vi "Att_Wobble.vi"(2 "Att Pos Z":refnum<vi>, 4 "Att Wobble End":dbl caption="End", 5 "Att Wobble Start":dbl caption="Start", 6 "Att Error":errorcluster, 7 "ourDLL":path, 8 "Att Wobble Stop2 2":refnum<vi>, 9 "Att DeviceHandle":u64) -> (0 "Att Error out":errorcluster, 3 "Att DeviceHandle out":u64)   [LabVIEW 2019]
panel:
  in  "Att Pos Z":dbl min=-500.0 max=3500.0 format="%#_7g"
  in  "Att Wobble Stop2":bool
  in  "Att Stop Wobble 2":bool
  in  "Att Stop Wobble":bool
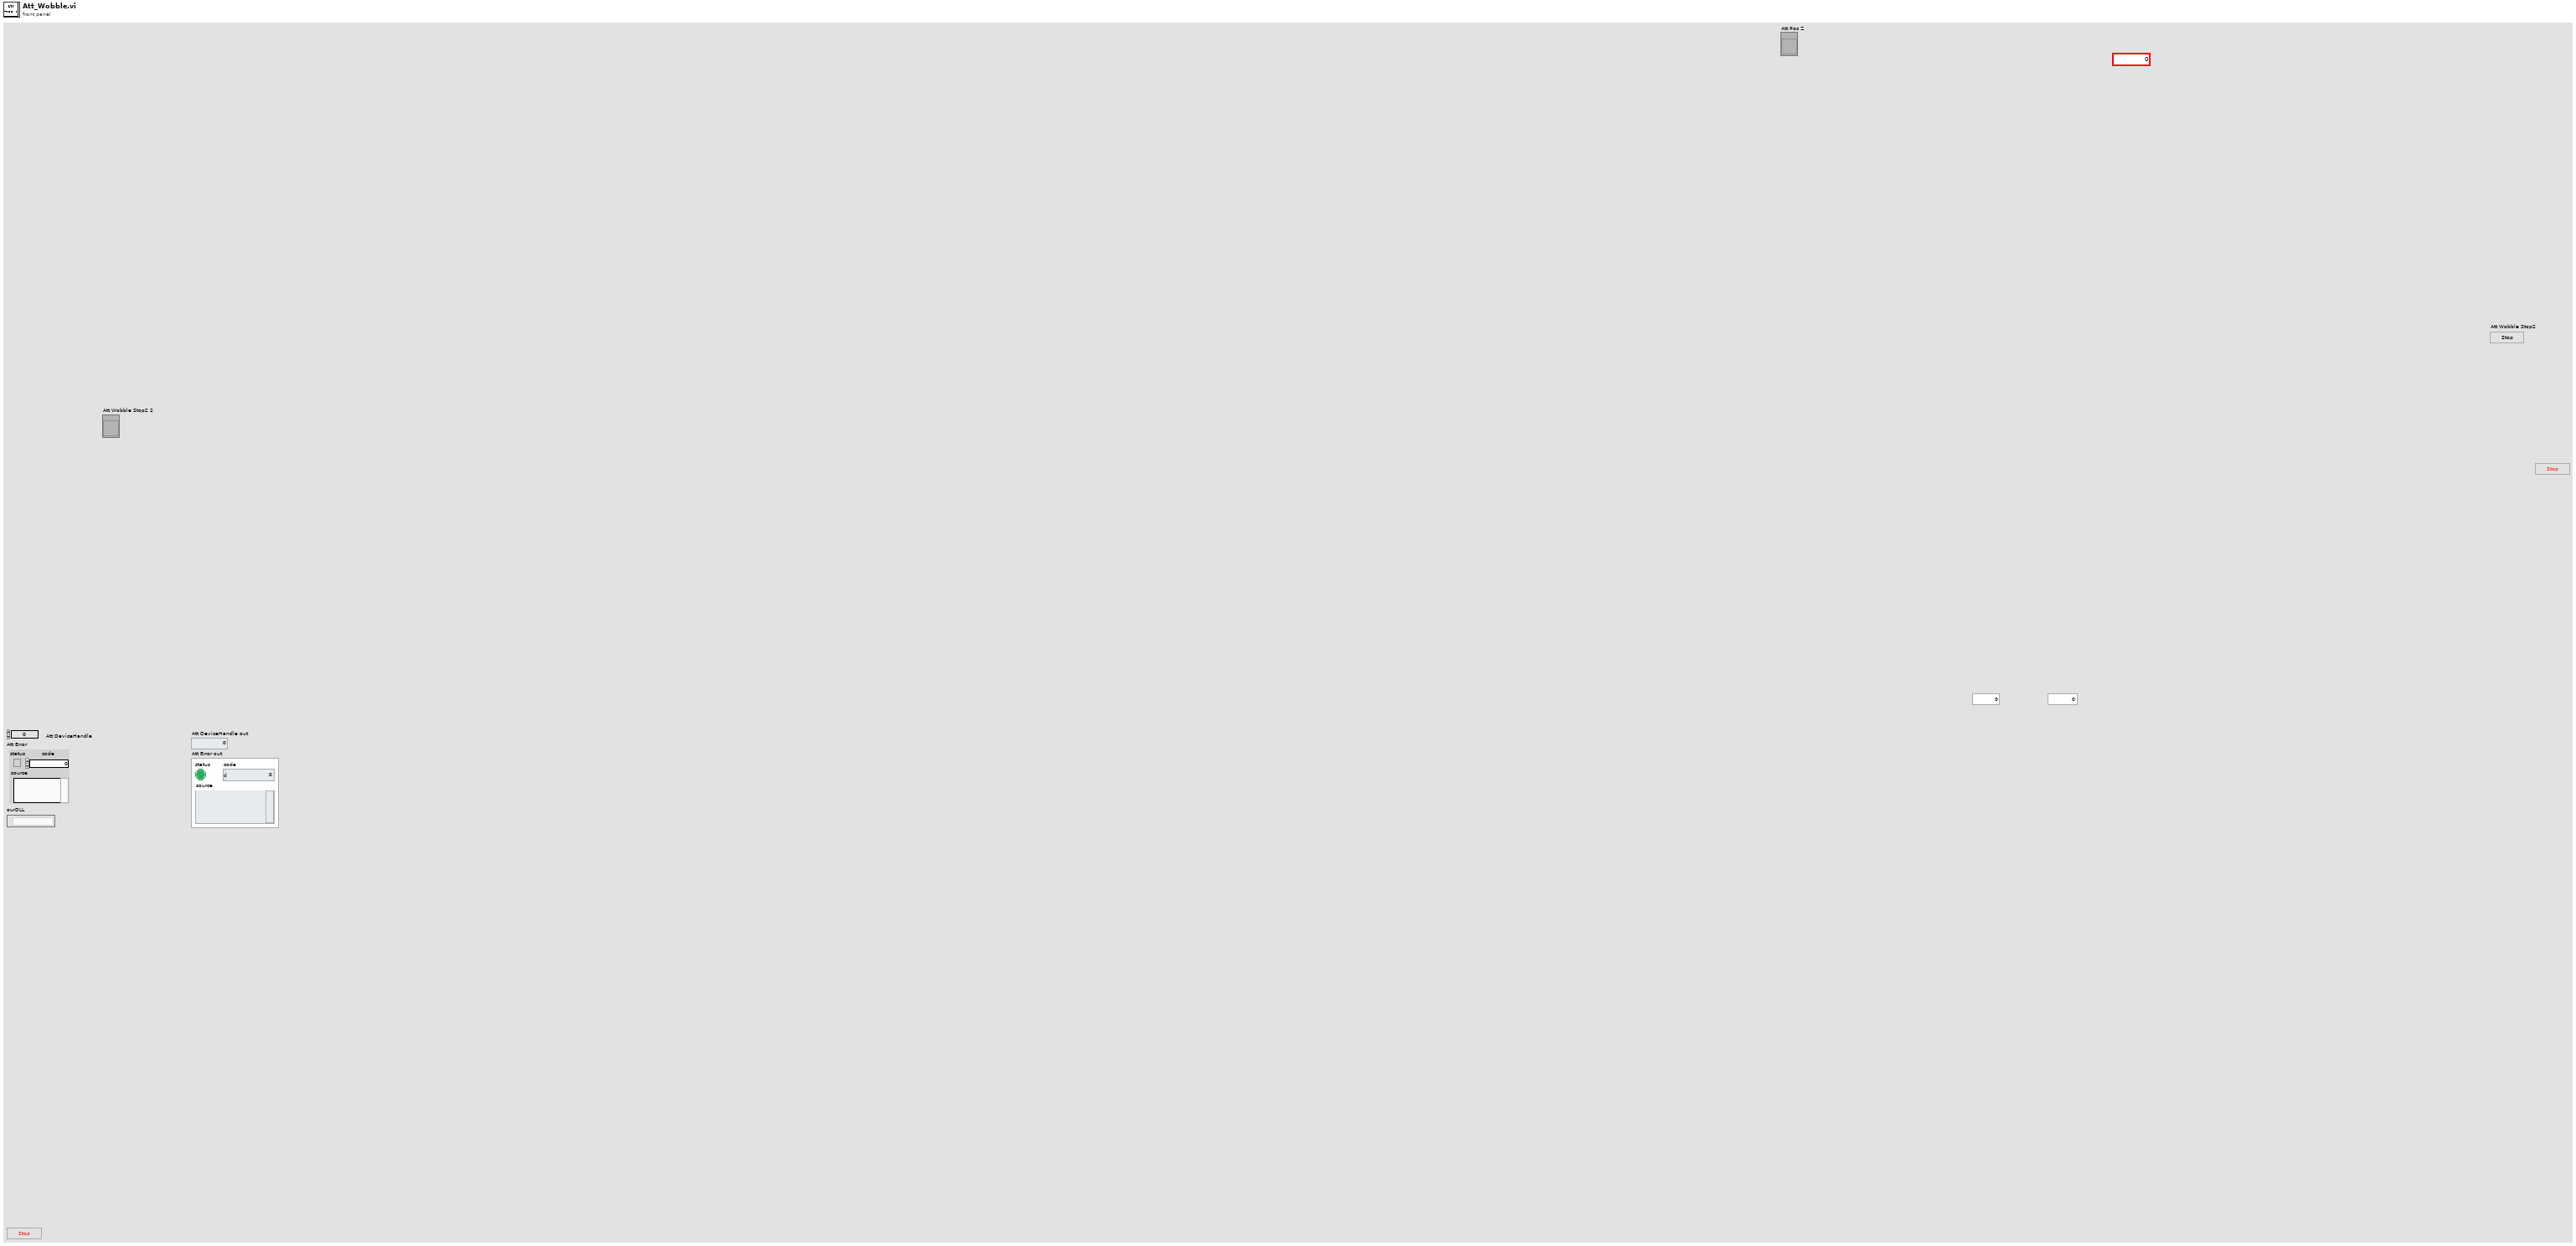
[diagram p1: front panel]
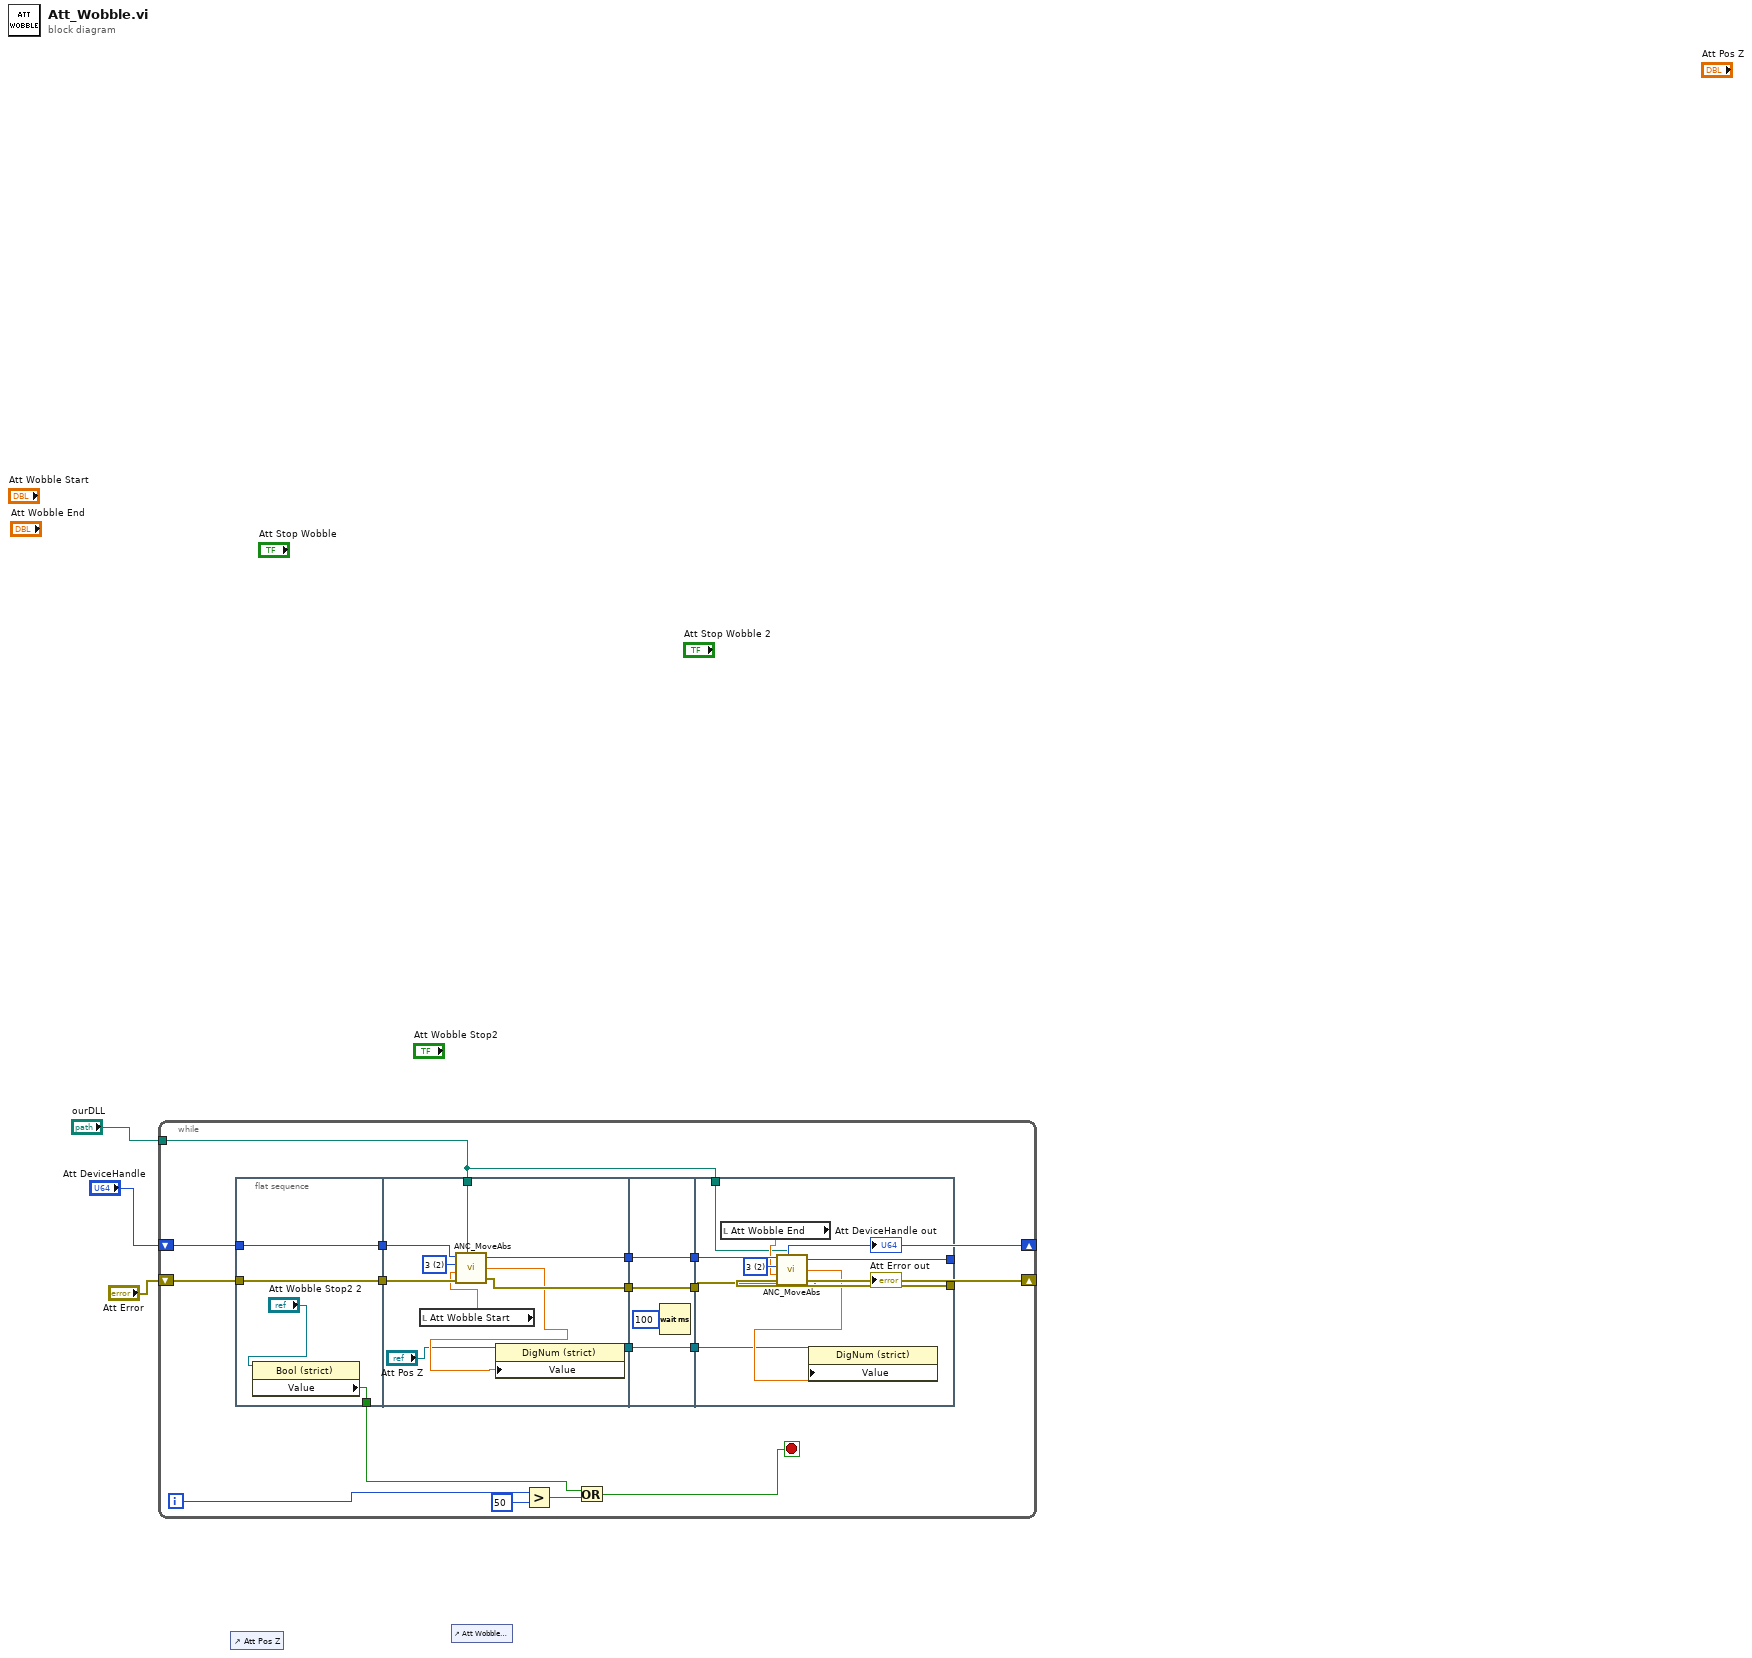
[diagram p0: block diagram]
diagram:
  n1 = while {
    shift-right: [w21] -> w2
    shift-left: "Att DeviceHandle" -> [w23]
    shift-right: [w20] -> w1
    shift-left: "Att Error" -> [w22]
    tunnel: "ourDLL" -> [w19]
    i -> [w18]
    stop <- w15 stop-if-true
    n2 = flat-sequence {
      tunnel: w22 -> [w26]
      tunnel: w23 -> [w27]
      tunnel: [w27] -> w8
      tunnel: [w26] -> w7
      tunnel: [w24] -> w6
      tunnel: [w37] -> w14
      tunnel: [w36] -> w12
      tunnel: w19 -> [w31]
      tunnel: [w29] -> w10
      tunnel: w8 -> [w34]
      tunnel: w7 -> [w33]
      tunnel: w14 -> [w41]
      tunnel: [w41] -> w13
      tunnel: w12 -> [w40]
      tunnel: [w40] -> w11
      tunnel: w10 -> [w39]
      tunnel: [w39] -> w9
      tunnel: w13 -> [w48]
      tunnel: w11 -> [w50]
      tunnel: w19 -> [w44]
      tunnel: w9 -> [w42]
      tunnel: [w49] -> w21
      tunnel: [w47] -> w20
      frame #0 {
        n3 = property class="Bool (strict)"(reference="Att Wobble Stop2 2") -> ("Value"=w24:bool)  [unwired: 1 in, 2 out]
      }
      frame #1 {
        w35 = u8 2 items=["1", "2", "3"] ("axis")
        n4 = local read "Att Wobble Start"() -> (w32:dbl)
        n5 = call "ANC_MoveAbs.vi"("Att DeviceHandle"=w34, "ourDLL"=w31, "axis"=w35, "Target pos"=w32, "Att Error"=w33) -> ("deviceHandle out"=w36:u64, "Out Position [µm | m°]"=w30:dbl, "error out"=w37:errorcluster)  [unwired: 1 in]
        n6 = property class="DigNum (strict)"(reference="Att Pos Z", "Value"=w30) -> (reference out=w29:refnum<vi>)  [unwired: 1 in, 1 out]
      }
      frame #2 {
        n7 = Wait (ms)(milliseconds to wait=u32 100) -> ()  [unwired: 1 out]
      }
      frame #3 {
        w46 = u8 2 items=["1", "2", "3"] ("axis")
        n8 = local read "Att Wobble End"() -> (w45:dbl)
        n9 = call "ANC_MoveAbs.vi"("Att DeviceHandle"=w50, "ourDLL"=w44, "axis"=w46, "Target pos"=w45, "Att Error"=w48) -> ("deviceHandle out"=w49:u64, "Out Position [µm | m°]"=w43:dbl, "error out"=w47:errorcluster)  [unwired: 1 in]
        n10 = property class="DigNum (strict)"(reference=w42, "Value"=w43) -> ()  [unwired: 1 in, 2 out]
      }
    }
    n11 = Greater?(x=w18, y=50) -> (0:w16:bool)
    n12 = Or(x=w6, y=w16) -> (x .or. y?=w15:bool)
  }
  "Att DeviceHandle out" <- w2
  "Att Error out" <- w1
  n13 = control-ref of="Att Pos Z"() -> ()  [unwired: 1 out]
  n14 = control-ref of="Att Wobble Stop2"() -> ()  [unwired: 1 out]
